vi "Instrument.Lockin.Client.vi"(8 "error in (no error)":errorcluster, 9 "Data":variant, 10 "Command":T1, 11 "Instrument.Lockin in":refnum<class "Instrument.Lockin.lvclass">) -> (0 "error out":errorcluster, 1 "Data out":variant, 3 "Instrument.Lockin out":refnum<class "Instrument.Lockin.lvclass">)   [LabVIEW 2016, in "Instrument.Lockin.lvclass"]
uses:
  Instrument.Lockin.lvclass
  C:/Program Files (x86)/National Instruments/LabVIEW 2016/user.lib/LevyLab/Levylab Instruments/SMOs/Instrument/Instrument.lvclass
  Typedefs/Instrument.Lockin.Commands--Enum.ctl
  <userlib>/LevyLab/Levylab Instruments/SMOs/Instrument/Instrument.lvclass
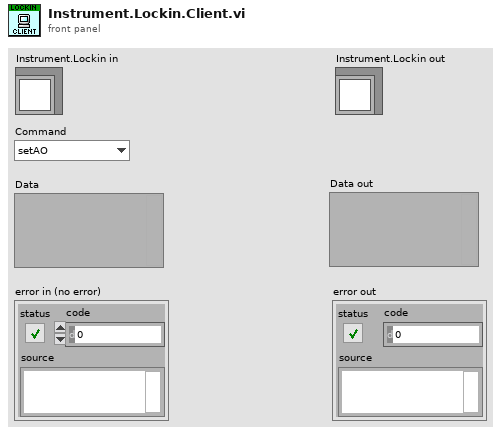
[diagram p1: front panel]
types:
  T1 = typedef "Instrument.Lockin.lvclass/Instrument.Lockin.Commands--Enum.ctl" = enum16{"setAO", "setAO_Amplitude", "setAO_DC", "setAO_Frequency", "setAO_Phase", "setAO_Function", "setAO_I+", "setREF", "setREF_Frequency", "setREF_Phase", "setIVmode", "Reset", "setSampling", "Trigger", "getAO", "getAI", "getResults", "getTrigger", "getIVmode", "getSampling", "getAOconfig", "getREFconfig", "setGain", "getGain", "setAutoSampling", "getAutoSampling", "setSweep", "getStatus", "getSweepResults", "getIVSweepResults", "startSweep", "stopSweep", "setAUX", "getAUX"}
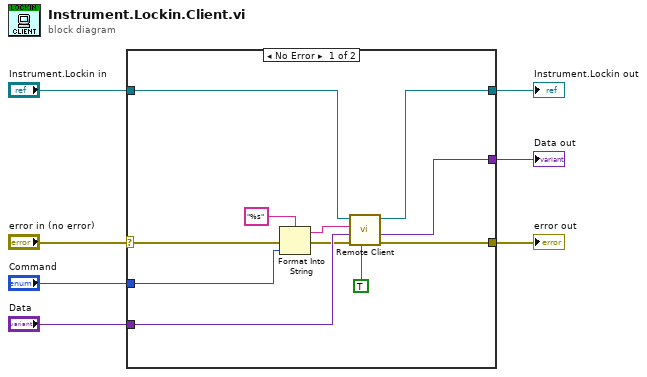
[diagram p0: block diagram]
diagram:
  n1 = case shown="No Error" "error in (no error)" {
    selector: "error in (no error)" -> [w11 w20]
    tunnel: "Data" -> [w18 _]
    tunnel: [w17 w20] -> w6
    tunnel: [w16 _] -> w5
    tunnel: "Command" -> [w15 _]
    tunnel: "Instrument.Lockin in" -> [w9 w19]
    tunnel: [w8 w19] -> w1
    frame No Error {
      n2 = Format Into String(format string="%s", error in=w11, w15) -> (resulting string=w10:string, error out=w13:errorcluster)  [unwired: 1 in]
      n3 = call <userlib>:"Remote Client.vi"("Wait for Response? [T]"=TRUE ("Wait for Response?"), "error in (no error)"=w13, "Data"=w18, "Command"=w10, "Instrument in"=w9) -> ("error out"=w17:errorcluster, "Data out"=w16:variant, "Instrument out"=w8:refnum<class "Instrument.Lockin.lvclass">)  [unwired: 3 in, 1 out]
    }
    frame Error {
    }
  }
  "Instrument.Lockin out" <- w1
  "error out" <- w6
  "Data out" <- w5
